vi "MH_ProcData_Modified_T2.vi"(10 "MH_DataProcThread_QRef":T3) -> ()   [LabVIEW 2023]
uses:
  Types/MH_DataProcThread_QRef.ctl
  Types/MH_DataProcThread_QData.ctl
  Types/MH_DataProcThread_QCmds.ctl
panel:
  out "element":T1={"Cmd"=enum."Proc", "nActual"=0, "Buffer"=[], "TickCount"=0, "Param"=0}
  out "output cluster":cluster{u64[], u32[]}
  out "T2 Data Array":u64[][](array[numeric])
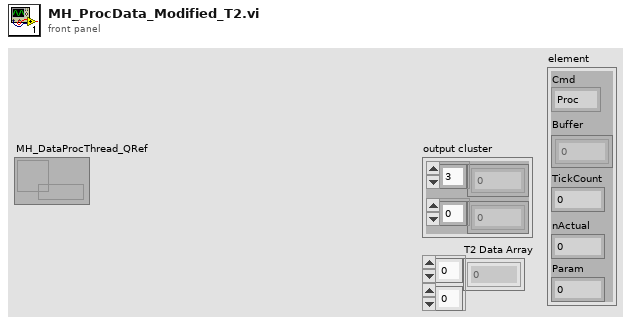
[diagram p1: front panel]
types:
  T1 = typedef "MH_DataProcThread_QData.ctl" = cluster{"Cmd":T2, "nActual":i32, "Buffer":u32[], "TickCount":u32, "Param":i32}
  T2 = typedef "MH_DataProcThread_QCmds.ctl" = enum16{"Exit", "Proc", "Init", "SetShift", "SetNumChannels", "SetHistAcqTime"}
  T3 = typedef "MH_DataProcThread_QRef.ctl" = refnum<queue>
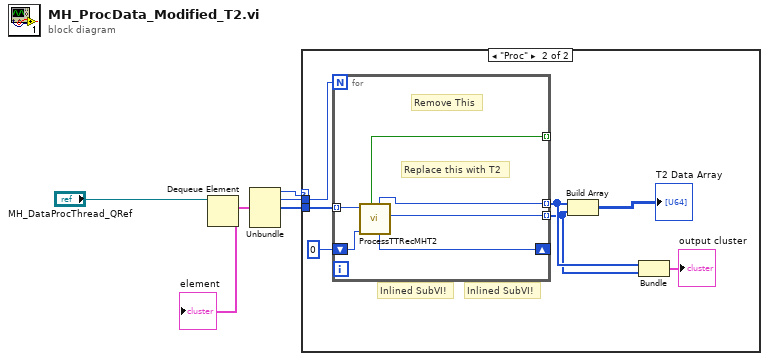
[diagram p0: block diagram]
diagram:
  n1 = Dequeue Element(queue="MH_DataProcThread_QRef") -> (element=w2:T1)  [unwired: 2 in, 3 out]
  "element" <- w2
  n2 = Unbundle(w2) -> ("Cmd"=w1:T2, "nActual"=w4:i32, "Buffer"=w3:u32[])  [unwired: 2 out]
  n3 = case shown="\"Proc\"" w1 {
    tunnel: w4 -> [_ w12]
    tunnel: w3 -> [_ w11]
    frame "Exit", Default {
    }
    frame "Proc" {
      # "Inlined SubVI!"
      # "Inlined SubVI!"
      n4 = for {
        N: w12 -> [_]
        tunnel: w11 -> [w16] mode=indexing
        shift-right: [w18] -> _
        shift-left: u64 0 ("oflcorr_out") -> [w17]
        tunnel: [w15] -> _ mode=indexing
        tunnel: [w14] -> w8 mode=indexing
        tunnel: [w13] -> w7 mode=indexing
        # "Replace this with T2"
        # "Remove This"
        n5 = call "ProcessTTRecMHT2.vi"("oflcorr_in"=w17, "rawbits"=w16) -> ("channel"=w13:u32, "oflcorr_out"=w18:u64, "timetag"=w14:u64, "is_photon"=w15:bool)  [unwired: 4 in, 2 out]
      }
      n6 = Build Array(w8, w7) -> (→"T2 Data Array":u64[][])
      n7 = Bundle(w8, w7) -> (→"output cluster":cluster{u64[], u32[]})  [unwired: 1 in]
    }
  }
